vi "Launch DQMH Tools by menu.vi"(5 "Project":string="Project", 7 "Application Instance":refnum<vi>, 8 "error in":errorcluster, 10 "Module Ref":refnum<vi>, 11 "DQMH Tools":T1) -> (0 "error out":errorcluster)   [LabVIEW 2019, in "Panther Dashboard.lvlib"]
doc: "Launch a DQMH scripting tool by typing one of the following strings in Quick Drop before pressing the Ctrl-Key shortcut for this plugin:\n\nCreate New DQMH Event - ae, new event, add event, create event, \"\" (empty string)\nRename DQMH Event - re, rename event\nRemove DQMH Event - rme, remove\nConvert DQMH Event - ce, convert\nAdd New DQMH Module - am, new mod, add mod, create mod\nRename DQMH Module - rm, rename module\nValidate DQMH Module - vm, validate\nCreate DQMH Module Template - ct, template\nCreate RT Tester - crt, rt\nNew DQMH Unit Test - cut, unit\n\nDefault Shortcut - [E]"
uses:
  Panther Dashboard.lvlib
  Shared/Shared.lvlib
  DQMH Tools Menu--enum.ctl
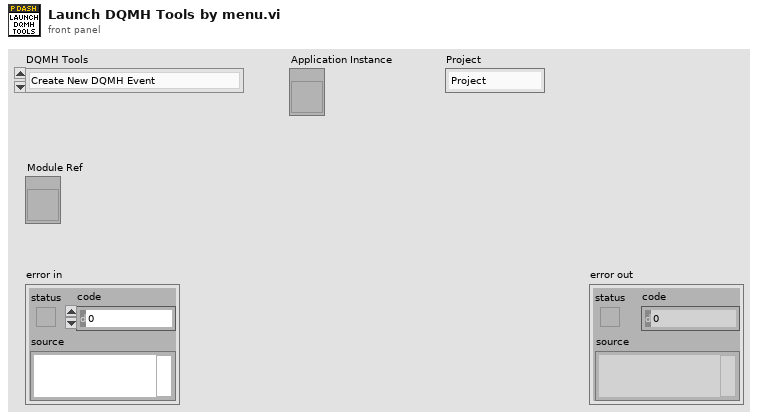
[diagram p1: front panel]
types:
  T1 = typedef "Panther Dashboard.lvlib/DQMH Tools Menu--enum.ctl" = enum16{"Create New DQMH Event", "Remove DQMH Event", "Convert DQMH Event", "Rename DQMH Event", "Add New DQMH Module", "Create RT Tester", "Rename DQMH Module", "Validate DQMH Module", "Create DQMH Module Template", "New DQMH  Unit Test"}
  T2 = enum32{"Invalid", "Standard", "Closed", "Hidden", "Minimized", "Maximized"}
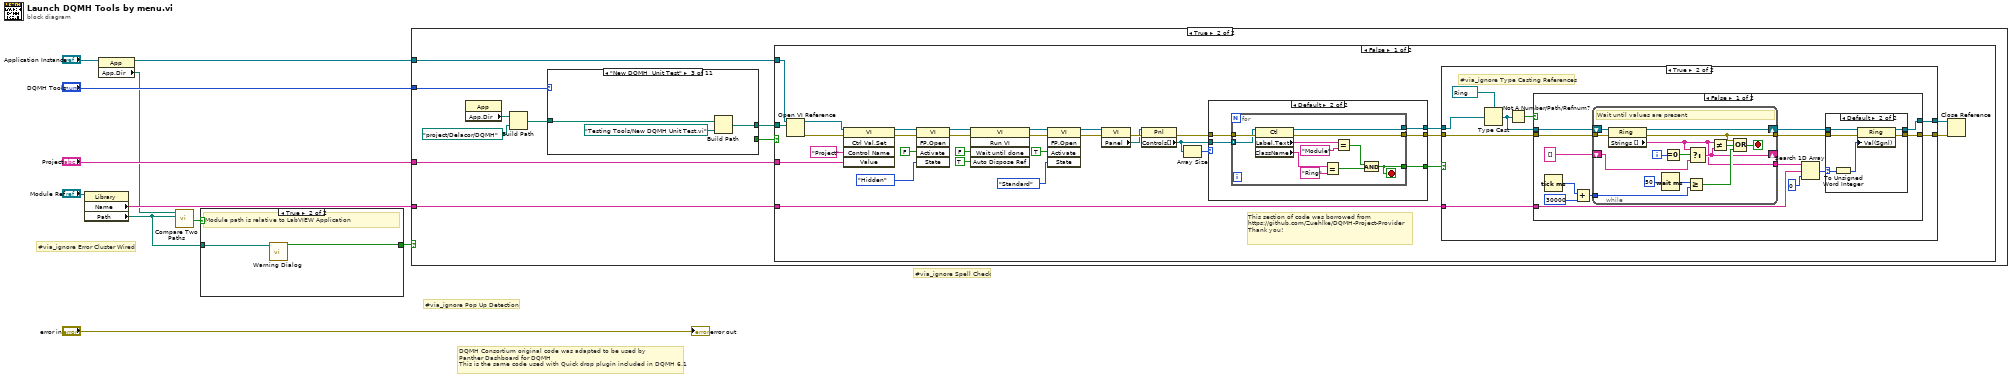
[diagram p0: block diagram]
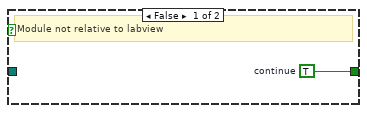
[diagram p2: hidden frame]
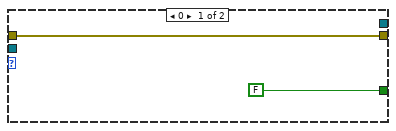
[diagram p4: hidden frame]
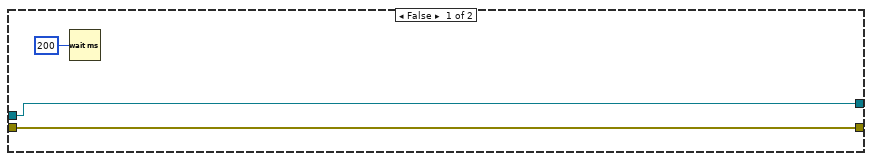
[diagram p5: hidden frame]
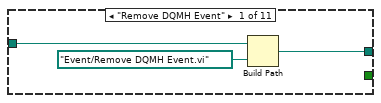
[diagram p9: hidden frame]
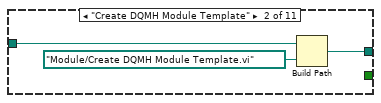
[diagram p10: hidden frame]
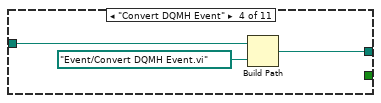
[diagram p11: hidden frame]
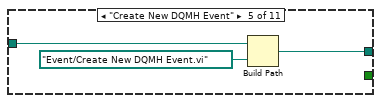
[diagram p12: hidden frame]
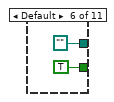
[diagram p13: hidden frame]
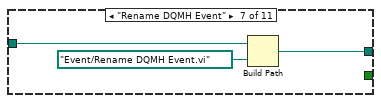
[diagram p14: hidden frame]
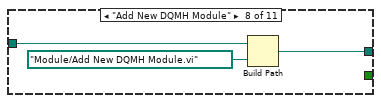
[diagram p15: hidden frame]
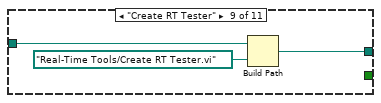
[diagram p16: hidden frame]
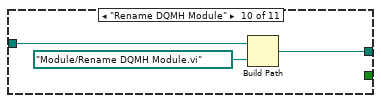
[diagram p17: hidden frame]
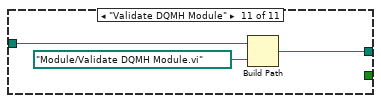
[diagram p18: hidden frame]
diagram:
  # "#via_ignore Error Cluster Wired"
  # "#via_ignore Pop Up Detection"
  # "#via_ignore Spell Check"
  # "DQMH Consortium original code was adapted to be used by \nPanther Dashboard for DQMH\nThis is the same code used with Quick drop plugin included in DQMH 6.1"
  n1 = property class="Library"(reference="Module Ref") -> ("Name"=w8:string, "Path"=w1:path)  [unwired: 1 in, 2 out]
  n2 = property class="App"(reference="Application Instance") -> (reference out=w4:refnum<vi>, "App.Dir"=w3:path)  [unwired: 1 in, 1 out]
  n3 = call <vilib>:"Compare Two Paths.vi"("Path 2"=w1, "Path 1"=w3) -> ("Path 2 Relative to Path 1?"=w2:bool)  [unwired: 6 in, 3 out]
  n4 = case shown="True" w2 {
    tunnel: [w12 w14] -> w6
    tunnel: w1 -> [_ w13]
    frame False {
      w12 = TRUE  # continue
      # "Module not relative to labview"
    }
    frame True {
      # "Module path is relative to LabVIEW Application"
      n5 = call "Warning Dialog.vi"("Path"=w13) -> ("Continue?"=w14:bool)  [unwired: 10 in]
    }
  }
  n6 = case shown="True" w6 {
    tunnel: "DQMH Tools" -> [_ w19]
    tunnel: "Project" -> [_ w17]
    tunnel: w4 -> [_ w16]
    tunnel: w8 -> [_ w15]
    frame False {
    }
    frame True {
      n7 = property class="App"() -> ("App.Dir"=w23:path)  [unwired: 2 in, 2 out]
      n8 = Build Path(base path=w23, name or relative path=path "project/Delacor/DQMH" ("Application:Directory Path")) -> (appended path=w21:path)
      n9 = case shown="\"New DQMH  Unit Test\"" w19 {
        tunnel: w21 -> [w125 w128 w131 w134 w137 _ w142 w145 w148 w151 w154]
        tunnel: [w124 w127 w130 w133 w136 path "" w141 w144 w147 w150 w153] -> w20
        tunnel: [_ _ _ _ _ TRUE _ _ _ _ _] -> w18
        frame "Remove DQMH Event" {
          n10 = Build Path(base path=w125, name or relative path=path "Event/Remove DQMH Event.vi") -> (appended path=w124:path)
        }
        frame "Create DQMH Module Template" {
          n11 = Build Path(base path=w128, name or relative path=path "Module/Create DQMH Module Template.vi") -> (appended path=w127:path)
        }
        frame "New DQMH  Unit Test" {
          n12 = Build Path(base path=w131, name or relative path=path "Testing Tools/New DQMH Unit Test.vi") -> (appended path=w130:path)
        }
        frame "Convert DQMH Event" {
          n13 = Build Path(base path=w134, name or relative path=path "Event/Convert DQMH Event.vi") -> (appended path=w133:path)
        }
        frame "Create New DQMH Event" {
          n14 = Build Path(base path=w137, name or relative path=path "Event/Create New DQMH Event.vi") -> (appended path=w136:path)
        }
        frame Default {
        }
        frame "Rename DQMH Event" {
          n15 = Build Path(base path=w142, name or relative path=path "Event/Rename DQMH Event.vi") -> (appended path=w141:path)
        }
        frame "Add New DQMH Module" {
          n16 = Build Path(base path=w145, name or relative path=path "Module/Add New DQMH Module.vi") -> (appended path=w144:path)
        }
        frame "Create RT Tester" {
          n17 = Build Path(base path=w148, name or relative path=path "Real-Time Tools/Create RT Tester.vi") -> (appended path=w147:path)
        }
        frame "Rename DQMH Module" {
          n18 = Build Path(base path=w151, name or relative path=path "Module/Rename DQMH Module.vi") -> (appended path=w150:path)
        }
        frame "Validate DQMH Module" {
          n19 = Build Path(base path=w154, name or relative path=path "Module/Validate DQMH Module.vi") -> (appended path=w153:path)
        }
      }
      n20 = case shown="False" w18 {
        tunnel: w20 -> [w41 _]
        tunnel: w17 -> [w33 _]
        tunnel: w16 -> [w32 _]
        tunnel: w15 -> [w24 _]
        frame False {
          # "This section of code was borrowed from\nhttps://github.com/Zuehlke/DQMH-Project-Provider\nThank you!"
          n21 = Open VI Reference(application reference (local)=w32, vi path=w41) -> (vi reference=w45:refnum<vi>, error out=w54:errorcluster)  [unwired: 4 in]
          n22 = invoke class="VI" method="Ctrl Val.Set"(reference=w45, error in=w54, "Control Name"="Project", "Value"=w33) -> (reference out=w43:refnum<vi>, error out=w53:errorcluster)  [unwired: 1 in, 3 out]
          n23 = invoke class="VI" method="FP.Open"(reference=w43, error in=w53, "Activate"=FALSE ("Wait Until Done"), "State"=T2."Hidden") -> (reference out=w39:refnum<vi>, error out=w52:errorcluster)  [unwired: 1 in, 3 out]
          n24 = invoke class="VI" method="Run VI"(reference=w39, error in=w52, "Wait until done"=FALSE ("Wait Until Done"), "Auto Dispose Ref"=TRUE ("Auto Dispose Reference")) -> (reference out=w36:refnum<vi>, error out=w51:errorcluster)  [unwired: 1 in, 3 out]
          n25 = invoke class="VI" method="FP.Open"(reference=w36, error in=w51, "Activate"=TRUE ("Activate?"), "State"=T2."Standard") -> (reference out=w25:refnum<vi>, error out=w46:errorcluster)  [unwired: 1 in, 3 out]
          n26 = property class="VI"(reference=w25, error in=w46) -> (error out=w49:errorcluster, "Panel"=w29:refnum<vi>)  [unwired: 1 out]
          n27 = property class="Pnl"(reference=w29, error in=w49) -> (error out=w48:errorcluster, "Controls[]"=w28:refnum<vi>[])  [unwired: 1 out]
          n28 = Array Size(array=w28) -> (size(s)=w27:i32)
          n29 = case shown="Default" w27 {
            tunnel: [_ w59] -> w26
            tunnel: [FALSE w58] -> w31
            tunnel: w48 -> [w56 w61]
            tunnel: [w56 w60] -> w47
            tunnel: w28 -> [_ w57]
            frame 0 {
            }
            frame Default {
              n30 = for {
                tunnel: w57 -> [w70] mode=indexing
                tunnel: [w69] -> w59
                tunnel: [w62] -> w58
                tunnel: w61 -> [w72]
                tunnel: [w71] -> w60
                stop <- w62 stop-if-true
                n31 = property class="Ctl"(reference=w70, error in=w72) -> (reference out=w69:refnum<vi>, error out=w71:errorcluster, "Label.Text"=w68:string, "ClassName"=w66:string)
                n32 = Equal?(x=w66, y="Ring" ("Class Name")) -> (x = y?=w63:bool)
                n33 = Equal?(x=w68, y="Module" ("Control Name")) -> (x = y?=w64:bool)
                n34 = Compound Arithmetic op=AND(w64, w63) -> (w62:bool)
              }
            }
          }
          n35 = case shown="True" w31 {
            tunnel: w26 -> [w74 w81]
            tunnel: w47 -> [w75 w83]
            tunnel: [w75 w82] -> w50
            tunnel: w24 -> [_ w79]
            tunnel: [w74 w76] -> w30
            frame False {
              n36 = Wait (ms)(milliseconds to wait=u32 200) -> ()  [unwired: 1 out]
            }
            frame True {
              # "#via_ignore Type Casting References"
              n37 = Type Cast(type=refnum<vi> refnum ("Module"), x=w81) -> (*(type *) &x=w78:refnum<vi>)
              n38 = Not A Number/Path/Refnum?(number/path/refnum=w78) -> (NaN/Path/Refnum?=w77:bool)
              n39 = case shown="False" w77 {
                tunnel: w83 -> [w97 w122]
                tunnel: w79 -> [w91 _]
                tunnel: [w89 w121] -> w76
                tunnel: w78 -> [w88 w121]
                tunnel: [w95 w122] -> w82
                frame False {
                  n40 = Tick Count (ms)() -> (millisecond timer value=w85:u32)
                  n41 = Add(x=w85, y=u32 30000) -> (x+y=w84:u32)
                  n42 = while {
                    tunnel: [w99] -> w92
                    shift-right: [w110] -> w90
                    shift-left: w88 -> [w109]
                    tunnel: w97 -> [w112]
                    tunnel: [w111] -> w96
                    shift-right: [w100] -> _
                    shift-left: string[] [] ("Strings []") -> [w104]
                    tunnel: w84 -> [w98]
                    i -> [w103]
                    stop <- w107 stop-if-true
                    # "Wait until values are present"
                    n43 = property class="Ring"(reference=w109, error in=w112) -> (reference out=w110:refnum<vi>, error out=w111:errorcluster, "Strings []"=w99:string[])
                    n44 = Wait (ms)(milliseconds to wait=u32 50) -> (millisecond timer value=w106:u32)
                    n45 = Equal To 0?(x=w103) -> (x = 0?=w102:bool)
                    n46 = Greater Or Equal?(x=w106, y=w98) -> (x >= y?=w108:bool)
                    n47 = Select(t=w99, s=w102, f=w104) -> (s? t:f=w100:string[])
                    n48 = Not Equal?(x=w99, y=w100) -> (x != y?=w101:bool)
                    n49 = Compound Arithmetic op=OR(w111, w101, w108) -> (w107:bool)
                  }
                  n50 = Search 1D Array(1D array=w92, element=w91, start index (0)=0) -> (index of element=w93:i32)
                  n51 = case shown="Default" w93 {
                    selector: w93 -> [_ w118]
                    tunnel: w90 -> [w113 w117]
                    tunnel: [w113 w115] -> w89
                    tunnel: w96 -> [w114 w120]
                    tunnel: [w114 w119] -> w95
                    frame -1 {
                    }
                    frame Default {
                      n52 = To Unsigned Word Integer(number=w118) -> (unsigned 16bit integer=w116:u16)
                      n53 = property class="Ring"(reference=w117, error in=w120, "Val(Sgnl)"=w116) -> (reference out=w115:refnum<vi>, error out=w119:errorcluster)
                    }
                  }
                }
                frame True {
                }
              }
            }
          }
          n54 = Close Reference(reference=w30, error in (no error)=w50) -> ()  [unwired: 1 out]
        }
        frame True {
        }
      }
    }
  }
  "error out" <- "error in"
